vi "Write GIF File Example.vi"(8 "error in (no error)":errorcluster) -> (0 "error out":errorcluster)   [LabVIEW 2011]
panel:
  out "x = y?":bool
  out "Array 2":u32[][](array[colorbox])
  in  "Array":u32[][][](array[colorbox])=array75x36x36[97200 elements]
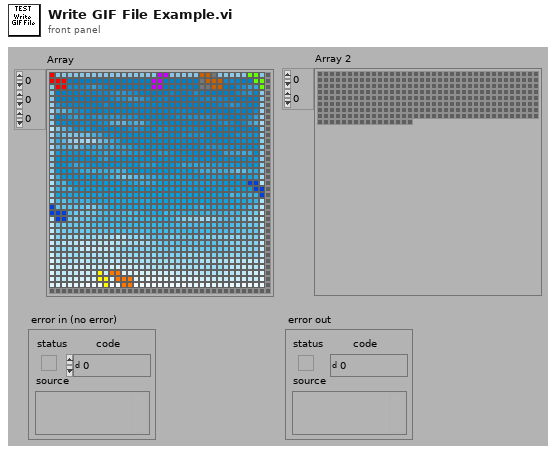
[diagram p1: front panel]
types:
  T1 = typedef "imagedata.ctl" = cluster{"image type":i32, "image depth":i32, "image":u8[], "mask":u8[], "colors":u32[], "Rectangle":cluster{"left":i16, "top":i16, "right":i16, "bottom":i16}}
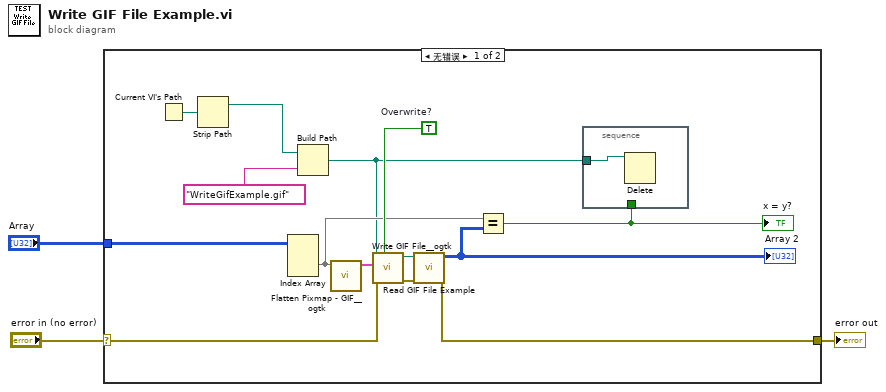
[diagram p0: block diagram]
diagram:
  n1 = case shown="无错误" "error in (no error)" {
    selector: "error in (no error)" -> [w17 w19]
    tunnel: [w9 w19] -> w2
    tunnel: "Array" -> [w6 _]
    frame No Error {
      w15 = TRUE  # Overwrite?
      n2 = Current VI's Path() -> (path=w12:path)
      n3 = Strip Path(path=w12) -> (stripped path=w11:path)  [unwired: 1 out]
      n4 = Index Array(array=w6) -> (element=w8:u32[][])  [unwired: 3 in]
      n5 = Build Path(base path=w11, name or relative path="WriteGifExample.gif") -> (appended path=w4:path)
      n6 = call <userlib>:"Flatten Pixmap - GIF__ogtk.vi"("PixelTable"=w8) -> ("image data"=w13:T1)  [unwired: 9 in, 1 out]
      n7 = call <userlib>:"Write GIF File__ogtk.vi"("overwrite? (false)"=w15, "error in (no error)"=w17, "image data"=w13, "path to GIF file"=w4) -> ("error out"=w14:errorcluster, "path"=w10:path)  [unwired: 6 in]
      n8 = call "Read GIF File Example.vi"("error in (no error)"=w14, "path to GIF file"=w10) -> ("error out"=w9:errorcluster, "Array"=w7:u32[][])  [unwired: 8 in]
      "Array 2" <- w7
      n9 = Equal?(x=w8, y=w7) -> (x = y?=w5:bool)
      "x = y?" <- w5
      n10 = stacked-sequence {
        tunnel: w5 -> [_]
        tunnel: w4 -> [w18]
        frame #0 {
          n11 = Delete(path (use dialog)=w18) -> ()  [unwired: 4 in, 3 out]
        }
      }
    }
    frame Error {
    }
  }
  "error out" <- w2
